vi "DAQ.vi"() -> ()   [LabVIEW 2020]
uses:
  <vilib>/MakerHub/LINX/Public/Peripherals/Digital/Digital Write 1 Chan.vi
  <vilib>/MakerHub/LINX/Public/Peripherals/Digital/Digital Read 1 Chan.vi
  <vilib>/MakerHub/LINX/Public/Peripherals/PWM/PWM Set Duty Cycle 1 Chan.vi
  <vilib>/MakerHub/LINX/Public/Peripherals/Analog/Analog Read 1 Chan.vi
  <vilib>/MakerHub/LINX/Public/Peripherals/Digital/Digital Write N Chans.vi
  <vilib>/MakerHub/LINX/Public/Peripherals/Digital/Digital Read N Chans.vi
  <vilib>/MakerHub/LINX/Public/Peripherals/Analog/Analog Read N Chans.vi
  <vilib>/MakerHub/LINX/Private/Local IO/LinxDigitalWrite.vi
  <vilib>/MakerHub/LINX/Public/Utilities/Check Channel.vi
  <vilib>/MakerHub/LINX/Private/Local IO/LinxDigitalRead.vi
  <vilib>/MakerHub/LINX/Private/Local IO/LinxAnalogRead.vi
  <vilib>/MakerHub/LINX/Public/Utilities/Open Serial.vi
  <vilib>/MakerHub/LINX/Private/Utilties/Generate Error.vi
  <vilib>/MakerHub/LINX/Public/Peripherals/PWM/PWM Set Duty Cycle N Chans.vi
  <vilib>/MakerHub/LINX/LMH-LINX.lvlib
panel:
  in  "Motor":bool
  out "AnalogREAD":dbl
  out "soil moisture":dbl(slide) scale=0.0..100.0
  out "Analog IN":dbl(graph)
  in  "Analog OUT":dbl(slide) scale=0.0..100.0
  out "DI Value":bool
  in  "Roof":bool
  in  "STOP":bool
  # "ANALOG I/O"
  # "DAQ\nUSING \nARDUINO"
  # "Digital OUT"
  # "DIGITAL I/O"
  # "Connect Arduino With Labview:\nTools -> Makehub-> LNIX -> LINX Firmware Wizard, then choose kind of Arduino and run this program."
  # "Digital IN"
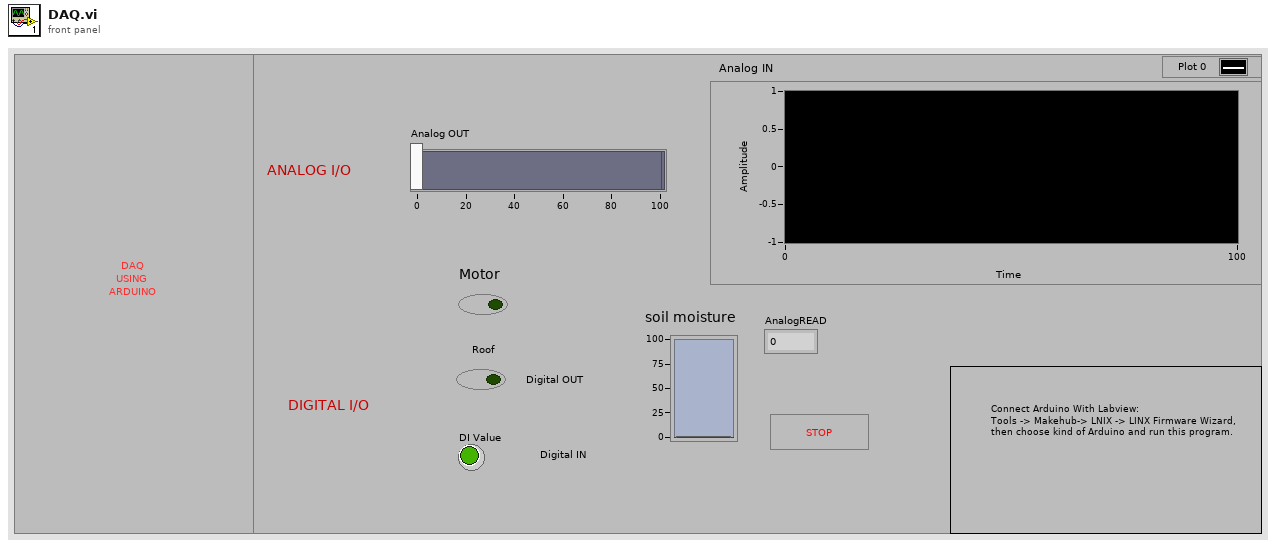
[diagram p1: front panel]
types:
  T1 = typedef "LMH-LINX.lvlib/LINX Ref.ctl" = cluster{"IO":T2, "Interface":T3, "LINX Device Config":T4}
  T2 = typedef "LMH-LINX.lvlib/Platform.ctl" = enum16{"Remote", "Local"}
  T3 = typedef "LMH-LINX.lvlib/Interface.ctl" = enum16{"Serial", "TCP"}
  T4 = typedef "LMH-LINX.lvlib/Device.lvlib/LINX Device Config.ctl" = cluster{"Interface":T3, "COM Port":refnum<visa-resource-name>, "TCP Configuration":T5, "Device Family":u8, "Device ID":u8, "Device Name":string, "TCP Ref":refnum<k5>, "Channels":T6}
  T5 = typedef "LMH-LINX.lvlib/Device.lvlib/TCP Config.ctl" = cluster{"IP Address":string, "Port":u16}
  T6 = typedef "LMH-LINX.lvlib/Channels.ctl" = cluster{"DI":u8[], "DO":u8[], "AI":u8[], "AO":u8[], "PWM":u8[], "QE":u8[], "UART":u8[], "I2C 2":u8[], "SPI":u8[], "CAN":u8[], "Servo":u8[], "AI Ref (V)":dbl, "AI Resolution (Bits)":u8, "AO Ref (V)":dbl, "AO Resolution (Bits)":u8}
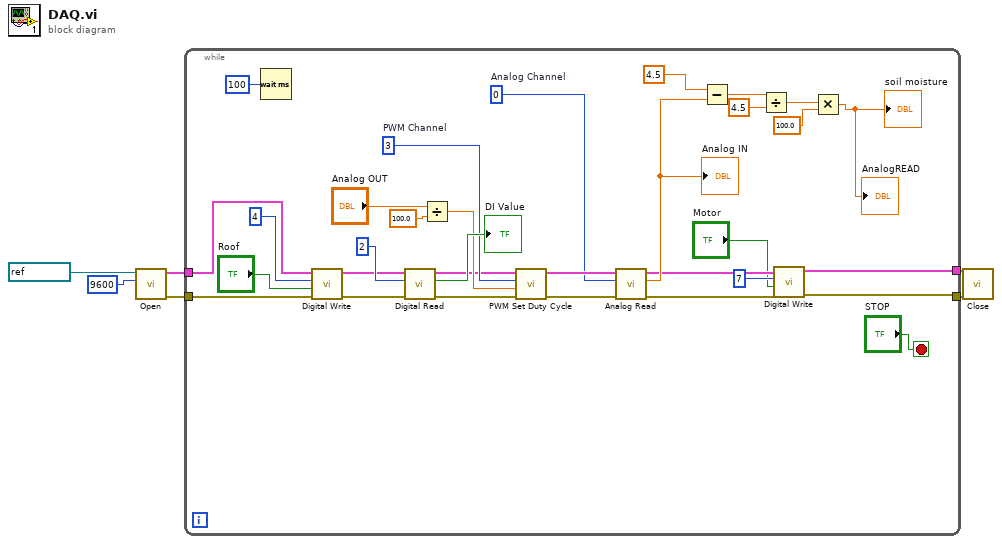
[diagram p0: block diagram]
diagram:
  n1 = call-poly <vilib>:"Open.vi"("Baud Rate Override"=u32 9600, "Serial Port"=refnum<visa-resource-name> "COM7") -> ("Error Out"=w4:errorcluster, "LINX Resource"=w3:T1)  [unwired: 7 in, 1 out]
  n2 = while {
    tunnel: w4 -> [w33]
    tunnel: w3 -> [w31]
    tunnel: [w9] -> w2
    tunnel: [w11] -> w1
    stop <- "STOP" stop-if-true
    w20 = u8 0  # Analog Channel
    w28 = u8 3  # PWM Channel
    n3 = Wait (ms)(milliseconds to wait=u32 100 ("millisecond timer value")) -> ()  [unwired: 1 out]
    n4 = call-poly <vilib>:"Digital Write.vi"("Error In"=w33, "Output Value"="Roof", "DO Channel"=u8 4, "LINX Resource"=w31) -> ("Error Out"=w29:errorcluster, "LINX Resource"=w30:T1)  [unwired: 6 in]
    n5 = call-poly <vilib>:"Digital Read.vi"("Error In"=w29, "DI Channel"=u8 2, "LINX Resource"=w30) -> ("Error Out"=w23:errorcluster, "DI Value"=→"DI Value":bool, "LINX Resource"=w24:T1)  [unwired: 6 in]
    n6 = Divide(x="Analog OUT", y=100.0) -> (x/y=w26:dbl)
    n7 = call-poly <vilib>:"PWM Set Duty Cycle.vi"("Error In"=w23, "Duty Cycle (0-1)"=w26, "PWM Channel"=w28, "LINX Resource"=w24) -> ("Error Out"=w21:errorcluster, "LINX Resource"=w22:T1)  [unwired: 6 in]
    n8 = call-poly <vilib>:"Analog Read.vi"("Error In"=w21, "Analog Channel"=w20, "LINX Resource"=w22) -> ("Error Out"=w10:errorcluster, "Voltage"=w19:dbl, "LINX Resource"=w12:T1)  [unwired: 5 in, 1 out]
    "Analog IN" <- w19
    n9 = Subtract(x=4.5, y=w19) -> (x-y=w17:dbl)
    n10 = Divide(x=w17, y=4.5) -> (x/y=w15:dbl)
    n11 = call-poly <vilib>:"Digital Write.vi"("Error In"=w10, "Output Value"="Motor", "DO Channel"=u8 7, "LINX Resource"=w12) -> ("Error Out"=w9:errorcluster, "LINX Resource"=w11:T1)  [unwired: 6 in]
    n12 = Multiply(x=w15, y=100.0) -> (x*y=→"soil moisture" →"AnalogREAD":dbl)
  }
  n13 = call <vilib>:"Close.vi"("Error In"=w2, "LINX Resource"=w1) -> ()  [unwired: 9 in, 1 out]
